vi "sv_Harmonic Magnitude and Phase (N Channels).vi"(0 "even-angle signals":cluster{"r0":dbl, "dr":dbl, "Y":dbl[]}[](array[cluster]) {"r0" format="%.2p"; "dr" format="%.2p"; "Y" format="%.2f"}, 2 "reset? (F)":bool, 5 "even-angle channel info":T7[](array[typedef]) {"channel info"."pregain" format="%.2f"; "channel info"."weighting filter" items=["Linear", "A-weighting", "B-weighting", "C-weighting", "ITU-R 468-4", "Dolby", "CCITT", "C-message", "Wb", "Wc", "Wd", "We", "Wf", "Wh", "Wj", "Wk", "Wm", "AES17 20 kHz lowpass", "AES17 40 kHz lowpass", "AES17 20 kHz highpass", "AES17 40 kHz highpass"]; "channel info"."dB reference" format="%^.1e"; "channel info"."engineering units" items=["custom..."=0, "V"=1, "A"=21, "C"=30, "pC"=31, "s"=32, "-"=29, "Pa"=2, "N"=20, "g"=3, "m/s^2"=4, "m/s"=5, "m"=6, "mm/s"=12, "mm"=13, "micron/s"=14, "micron"=15, "in/s^2"=7, "in/s"=8, "in"=9, "mil/s"=10, "mil"=11, "rad/s^2"=16, "rad/s"=17, "rad"=18, "deg/s^2"=26, "deg/s"=27, "deg"=28, "RPM"=22, "cycle/s^2"=23, "Hz"=24, "cycle"=25, "strain"=19]; "channel info"."sensor sensitivity" format="%#_5f"}, 7 "even-angle position info":T9, 9 "orders to compute (1.0)":dbl[](array[numeric])=[1.0] format="%.2f", 11 "error in (no error)":errorcluster, 12 "bandwidth [order]":dbl=1.0 format="%.2f", 14 "zero delay? (F)":bool) -> (4 "magnitudes [RMS]":T11(array[cluster]) {"magnitude" format="%.2f"; "time/rev/freq" format="%.2f"}, 6 "phases [phase lag]":T10(array[cluster]) {"phase" format="%.2f"; "time/rev/freq" format="%.2f"}, 10 "magnitudes info":T1[](array[typedef]) {"x-axis units" items=["Time (s)"=0, "Frequency-CB (Hz)"=1, "Frequency-CPB (Hz)"=1248, "Frequency-Arbitrary (Hz)"=2357, "Quefrency (s)"=2, "Revolutions (rev)"=3, "Order"=4, "Speed (RPM)"=11, "Speed (rad/s)"=21, "Index"=65535]; "weighting filter" items=["Linear", "A-weighting", "B-weighting", "C-weighting", "ITU-R 468-4", "Dolby", "CCITT", "C-message", "Wb", "Wc", "Wd", "We", "Wf", "Wh", "Wj", "Wk", "Wm", "AES17 20 kHz lowpass", "AES17 40 kHz lowpass", "AES17 20 kHz highpass", "AES17 40 kHz highpass"]; "dB reference [EU]" format="%.2f"; "engineering units" items=["custom..."=0, "V"=1, "A"=21, "C"=30, "pC"=31, "s"=32, "-"=29, "Pa"=2, "N"=20, "g"=3, "m/s^2"=4, "m/s"=5, "m"=6, "mm/s"=12, "mm"=13, "micron/s"=14, "micron"=15, "in/s^2"=7, "in/s"=8, "in"=9, "mil/s"=10, "mil"=11, "rad/s^2"=16, "rad/s"=17, "rad"=18, "deg/s^2"=26, "deg/s"=27, "deg"=28, "RPM"=22, "cycle/s^2"=23, "Hz"=24, "cycle"=25, "strain"=19]; "spectral info"."window" items=["None "=0, "Hanning"=1, "Hamming"=2, "Blackman-Harris"=3, "Exact Blackman"=4, "Blackman"=5, "Flat Top"=6, "4 Term B-Harris "=7, "7 Term B-Harris"=8, "Low Sidelobe"=9, "Force - Exponential"=10, "Gaussian"=62]}, 15 "error out":errorcluster)   [LabVIEW 2017, in "SoundVib_ContSweptSine.lvlib"]
doc: "Computes the magnitudes and phases of designated orders in an even-angle signal. The data type you wire to the <B>even-angle signal</B> input or the <B>order waveforms [EU]</B> input determines the polymorphic instance to use."
uses:
  <vilib>/addons/Sound and Vibration/svt_Continuous Swept Sine/SoundVib_ContSweptSine.lvlib
  <vilib>/addons/Sound and Vibration/Order Analysis/Misc/OAT Position Info.ctl
  <vilib>/addons/_NISVFA/_Shared subVIs/Controls/svc_Resampled Channel Info.ctl
  <vilib>/addons/_NISVFA/_Shared subVIs/Controls/svc_Channel Info.ctl
  <vilib>/addons/_NISVFA/_Shared subVIs/Controls/svc_Engineering Units Text Ring.ctl
  <vilib>/addons/_NISVFA/_Shared subVIs/Controls/svc_Weighting Filter Text Ring.ctl
  <vilib>/addons/_NISVFA/_Shared subVIs/Controls/svc_Spectrum Info.ctl
  <vilib>/addons/_NISVFA/_Shared subVIs/Controls/svc_X-Axis Units.ctl
  <vilib>/addons/_NISVFA/_Shared subVIs/Controls/svc_Spectrum Type.ctl
  <vilib>/addons/_NISVFA/_Shared subVIs/Controls/svc_Complimentary Spectrum Units.ctl
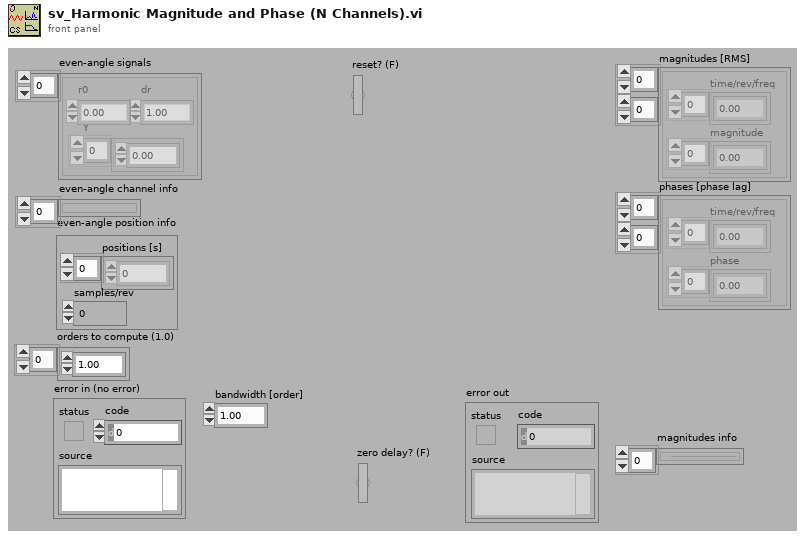
[diagram p1: front panel]
types:
  T1 = typedef "svc_Spectrum Info.ctl" = cluster{"channel name":string, "description":string, "x-axis units":T2, "spectral info":cluster{"spectrum type":T3, "linear/dB":enum16{"linear", "dB"}, "window":u16, "window size":i32, "FFT size":i32}, "engineering units":T4, "custom label":string, "dB reference [EU]":dbl, "peak units":enum16{"rms", "peak", "peak-peak"}, "weighting filter":T5, "spectral density?":bool, "unit label":string, "spectrum skewed?":bool, "complimentary spectrum units":T6}
  T2 = typedef "svc_X-Axis Units.ctl" = u16
  T3 = typedef "svc_Spectrum Type.ctl" = enum16{"FFT Spectrum [complex]", "Amplitude [Magnitude]", "Power [Magnitude^2]", "Cross Spectrum [complex]", "Frequency Response [Complex]"}
  T4 = typedef "svc_Engineering Units Text Ring.ctl" = u16
  T5 = typedef "svc_Weighting Filter Text Ring.ctl" = u16
  T6 = typedef "svc_Complimentary Spectrum Units.ctl" = enum16{"none", "radians", "degrees", "cycles", "imaginary"}
  T7 = typedef "svc_Resampled Channel Info.ctl" = cluster{"channel name":string, "description":string, " channel info":T8}
  T8 = typedef "svc_Channel Info.ctl" = cluster{"sensor sensitivity":dbl, "engineering units":T4, "dB reference":dbl, "custom label":string, "weighting filter":T5, "pregain":dbl}
  T9 = typedef "OAT Position Info.ctl" = cluster{"positions [s]":dbl[], "samples/rev":dbl}
  T10 = cluster{"time/rev/freq":dbl[], "phase":dbl[]}[][]
  T11 = cluster{"time/rev/freq":dbl[], "magnitude":dbl[]}[][]
  T12 = cluster{"dB on? (F)":bool, "unwrap phase? (T)":bool, "unit in degree? (T)":bool}
  T13 = cluster{"bandwidth [order] out":dbl, "stop band attenuation":u16}
  T14 = cluster{"unwrap phase? (T)":bool, "unit in degree? (T)":bool}
  T15 = typedef "SoundVib_TachProcess.lvlib/speed profile.ctl" = cluster{"time [s]":dbl[], "speed [RPM]":dbl[]}
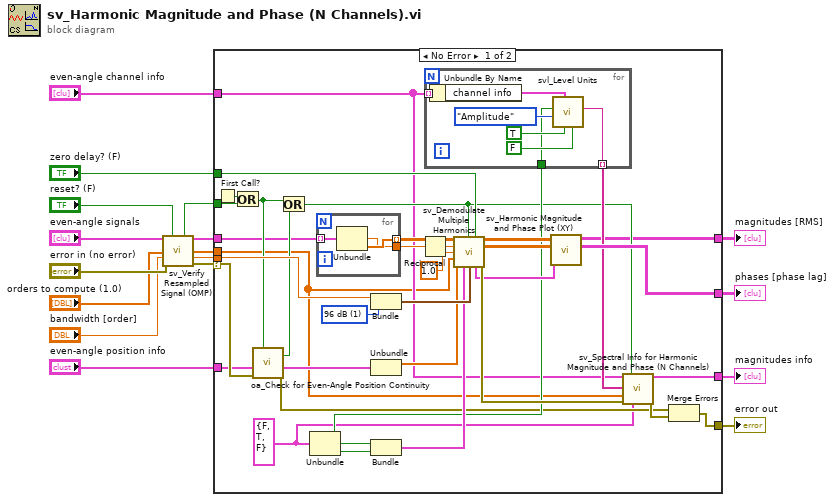
[diagram p0: block diagram]
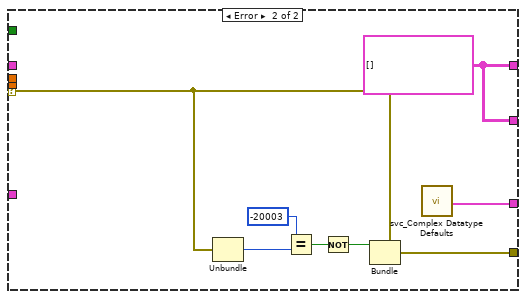
[diagram p2: hidden frame]
diagram:
  n1 = call <vilib>:"sv_Verify Resampled Signal (OMP).vi"("resampled signal"="even-angle signals", "reset in (T)"="reset? (F)", "orders to compute (1.0)"="orders to compute (1.0)", "bandwidth [order]"="bandwidth [order]", "error in (no error)"="error in (no error)") -> ("reset out (T)"=w7:bool, "resampled signal out"=w10:cluster{"r0":dbl, "dr":dbl, "Y":dbl[]}[], "orders to compute (1.0) out"=w3:dbl[], "bandwidth [order] out"=w5:dbl, "error out"=w9:errorcluster)  [unwired: 2 in, 4 out]
  n2 = case shown="No Error" w9 {
    selector: w9 -> [w26 w68]
    tunnel: "even-angle position info" -> [w22 _]
    tunnel: [w53 w71] -> w16
    tunnel: [w20 w71] -> w15
    tunnel: w7 -> [w36 _]
    tunnel: [w32 w65] -> w14
    tunnel: "even-angle channel info" -> [w24 _]
    tunnel: [w52 w64] -> w12
    tunnel: w10 -> [w23 _]
    tunnel: w5 -> [w35 _]
    tunnel: w3 -> [w19 _]
    tunnel: "zero delay? (F)" -> [w30 _]
    frame No Error {
      w18 = T12 {"dB on? (F)"=FALSE, "unwrap phase? (T)"=TRUE, "unit in degree? (T)"=FALSE} ("view")
      w42 = u16 1 items=["72 dB", "96 dB", "120 dB"] ("stop band attenuation")
      n3 = First Call?() -> (First Call?: T/F=w37:bool)
      n4 = Or(x=w37, y=w36) -> (x .or. y?=w29:bool)
      n5 = call <vilib>:"oa_Check for Even-Angle Position Continuity.vi"("reset in"=w29, "error in (no error)"=w26, "even-angle position info"=w22) -> ("error out"=w25:errorcluster, "even-angle position info dup"=w21:T9, "position not continuous"=w28:bool)  [unwired: 6 out]
      n6 = Or(x=w29, y=w28) -> (x .or. y?=w27:bool)
      n7 = Unbundle(w18) -> ("dB on? (F)"=w34:bool, "unwrap phase? (T)"=w39:bool, "unit in degree? (T)"=w33:bool)
      n8 = for {
        tunnel: w23 -> [w56] mode=indexing
        tunnel: [w55] -> w47 mode=indexing
        tunnel: [w54] -> w48
        n9 = Unbundle(w56) -> ("dr"=w54:dbl, "Y"=w55:dbl[])  [unwired: 1 out]
      }
      n10 = Bundle("bandwidth [order] out"=w35, "stop band attenuation"=w42) -> (w43:T13)  [unwired: 1 out]
      n11 = Unbundle(w21) -> ("positions [s]"=w40:dbl[])  [unwired: 1 out]
      n12 = Bundle("unwrap phase? (T)"=w39, "unit in degree? (T)"=w33) -> (w38:T14)  [unwired: 1 out]
      n13 = Reciprocal(x=w48) -> (1/x=w46:dbl)
      n14 = for {
        tunnel: w24 -> [w62] mode=indexing
        tunnel: [w60] -> w44 mode=indexing
        tunnel: w34 -> [w57]
        n15 = Unbundle By Name(w62) -> ("channel info"=w61:T8)
        n16 = call <vilib>:"svl_Level Units.vi"("include weighting if dB On FALSE"=FALSE, "rms level (T)"=TRUE, "channel info"=w61, "view mode"=enum16{"Power", "Amplitude"}."Amplitude", "dB On (T)"=w57) -> ("unit label"=w60:string)  [unwired: 1 in, 5 out]
      }
      n17 = call <vilib>:"sv_Demodulate Multiple Harmonics.vi"("Y"=w47, "reset? (True)"=w27, "zero delay? (F)"=w30, "samples/rev"=w46, "samples/rev wanted"=1.0 ("x"), "orders (1.0)"=w19, "time stamps in"=w40, "phase setting"=w38, "order info"=w43) -> ("magnitudes (RMS)"=w51:dbl[][][], "phase lag"=w50:dbl[][][], "speed profile"=w41:T15, "error out"=w45:errorcluster)  [unwired: 3 out]
      n18 = call <vilib>:"sv_Harmonic Magnitude and Phase Plot (XY).vi"("speed profile"=w41, "phase lag  (even angular)"=w50, "magnitudes (even angular)"=w51) -> ("phase lag"=w53:cluster{"X":dbl[], "Y":dbl[]}[][], "magnitudes"=w20:cluster{"X":dbl[], "Y":dbl[]}[][])  [unwired: 3 in, 4 out]
      n19 = call <vilib>:"sv_Spectral Info for Harmonic Magnitude and Phase (N Channels).vi"("channel info"=w24, "reset? (T)"=w27, "unit labels"=w44, "orders to compute"=w19, "error in (no error)"=w45, "view"=w18) -> ("spectrum info"=w52:T1[], "error out"=w31:errorcluster)  [unwired: 8 in]
      n20 = Merge Errors(w25, w31) -> (w32:errorcluster)
    }
    frame Error {
      w71 = cluster{"X":dbl[], "Y":dbl[]}[][] [] ("magnitudes")
      n21 = Unbundle(w68) -> ("code"=w70:i32)  [unwired: 2 out]
      n22 = Equal?(x=-20003 ("t"), y=w70) -> (x = y?=w67:bool)
      n23 = Not(x=w67) -> (.not. x?=w66:bool)
      n24 = Bundle(cluster=w68, "status"=w66) -> (w65:errorcluster)  [unwired: 2 out]
      n25 = call <vilib>:"svc_Complex Datatype Defaults.vi"() -> ("empty array of spectrum info"=w64:T1[])  [unwired: 19 out]
    }
  }
  "magnitudes [RMS]" <- w15
  "phases [phase lag]" <- w16
  "error out" <- w14
  "magnitudes info" <- w12
